vi "Create Listbox IP Text - Multi FPGA.vi"(8 "error in (no error)":errorcluster, 10 "rios and analog replays":T1(array[cluster]), 11 "Section Ref in":T2 format="%.0x") -> (0 "error out":errorcluster, 2 "listbox text":string[][](array[string]), 3 "Section Ref out":T2 format="%.0x", 5 "not present item indexes":i32[](array[numeric]))   [LabVIEW 2015, in "Engine Simulation Toolkit System Explorer.lvlib"]
uses:
  Engine Simulation Toolkit System Explorer.lvlib
  <vilib>/NI Veristand/Custom Device API/Custom Device Item Ref.ctl
  Shared/Properties.vi
  Shared/Constants and GUIDs.vi
  <vilib>/NI Veristand/Custom Device API/Get Item Property (String).vi
  <vilib>/NI Veristand/Custom Device API/Custom Device API.lvlib
  Shared/Engine Simulation Toolkit Shared.lvlib
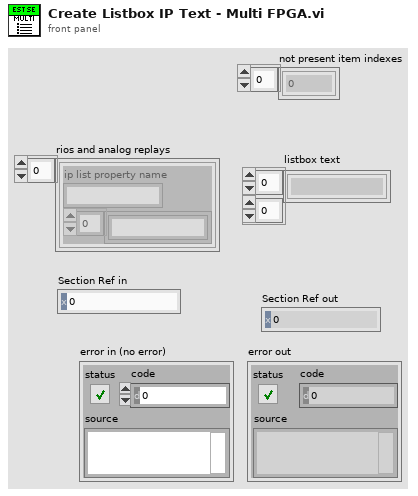
[diagram p1: front panel]
types:
  T1 = cluster{"ip list property name":string, string[]}[]
  T2 = typedef "Custom Device API.lvlib/Custom Device Item Ref.ctl" = u64
  T3 = typedef "Custom Device API.lvlib/Custom Device Item Info.ctl" = cluster{"Name":string, "Is Channel":bool, "GUID":string, "Is Waveform":bool}
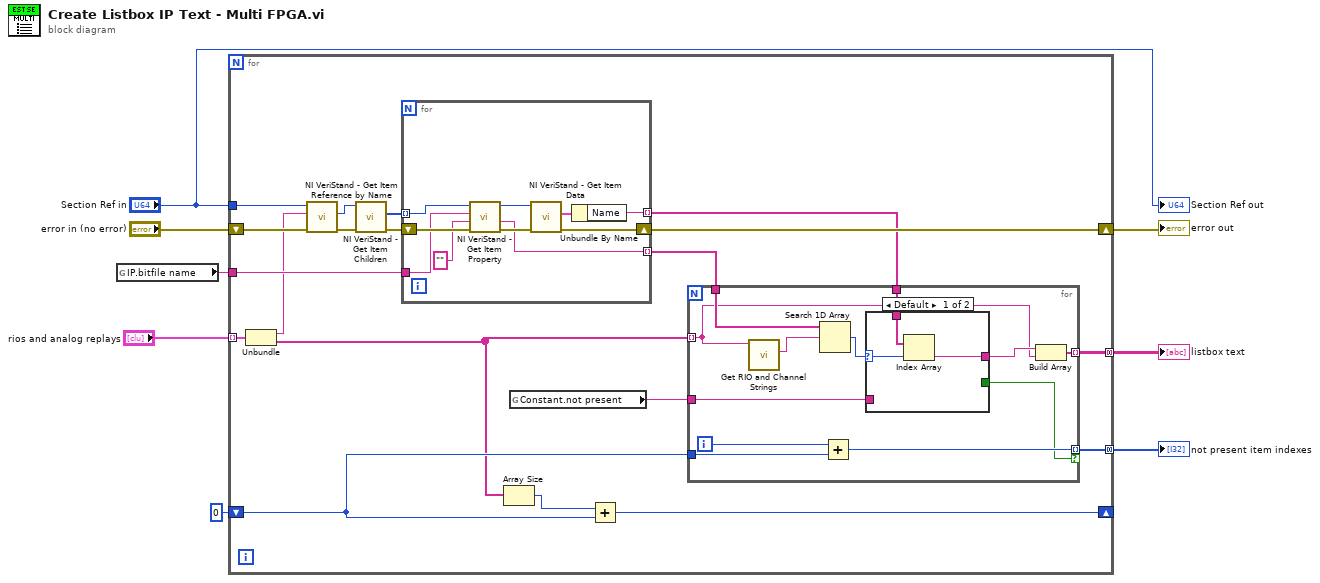
[diagram p0: block diagram]
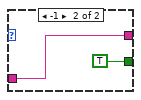
[diagram p2: hidden frame]
diagram:
  n1 = global read "Properties.vi" "IP.bitfile name"() -> (w8:string)
  n2 = for {
    tunnel: w8 -> [w27]
    tunnel: "rios and analog replays" -> [w18] mode=indexing
    tunnel: [w21] -> w7 mode=concatenating
    tunnel: [w24] -> w6 mode=concatenating
    shift-right: [w26] -> w1
    shift-left: "error in (no error)" -> [w16]
    shift-right: [w20] -> _
    shift-left: 0 -> [w19]
    tunnel: "Section Ref in" -> [w15]
    n3 = Unbundle(w18) -> ("ip list property name"=w14:string, w9:string[])
    n4 = call <vilib>:"NI VeriStand - Get Item Reference by Name.vi"("error in (no error)"=w16, "Item Name"=w14, "Parent Ref in"=w15) -> ("error out"=w17:errorcluster, "Item Ref"=w11:T2)  [unwired: 5 in, 2 out]
    n5 = call <vilib>:"NI VeriStand - Get Item Children.vi"("error in (no error)"=w17, "Item Ref in"=w11) -> ("error out"=w22:errorcluster, "Child Refs"=w23:T2[])  [unwired: 6 in, 2 out]
    n6 = for {
      shift-right: [w49] -> w26
      shift-left: w22 -> [w54]
      tunnel: w23 -> [w52] mode=indexing
      tunnel: w27 -> [w51]
      tunnel: [w46] -> w13 mode=indexing
      tunnel: [w45] -> w12 mode=indexing
      n7 = call-poly <vilib>:"NI VeriStand - Get Item Property.vi"("error in (no error)"=w54, "Default Value"="", "Property Name"=w51, "Item Ref in"=w52) -> ("error out"=w53:errorcluster, "Value"=w46:string, "Item Ref out"=w48:T2)  [unwired: 4 in, 1 out]
      n8 = call <vilib>:"NI VeriStand - Get Item Data.vi"("error in (no error)"=w53, "Item Ref in"=w48) -> ("error out"=w49:errorcluster, "Item Info"=w47:T3)  [unwired: 6 in, 2 out]
      n9 = Unbundle By Name(w47) -> ("Name"=w45:string)
    }
    n10 = Array Size(array=w9) -> (size(s)=w10:i32)
    n11 = global read "Constants and GUIDs.vi" "Constant.not present"() -> (w25:string)
    n12 = Add(x=w10, y=w19) -> (x+y=w20:i32)
    n13 = for {
      tunnel: w9 -> [w29] mode=indexing
      tunnel: w13 -> [w39]
      tunnel: w12 -> [w37]
      tunnel: [w35] -> w21 mode=indexing
      tunnel: w25 -> [w34]
      tunnel: [w31] -> w24 mode=indexing if=w30
      tunnel: w19 -> [w32]
      i -> [w33]
      n14 = call "Get RIO and Channel Strings.vi"("rio/channel"=w29) -> ("channel"=w28:string)  [unwired: 9 in, 1 out]
      n15 = Search 1D Array(1D array=w39, element=w28) -> (index of element=w38:i32)  [unwired: 1 in]
      n16 = Add(x=w33, y=w32) -> (x+y=w31:i32)
      n17 = case shown="Default" w38 {
        selector: w38 -> [w41 _]
        tunnel: [w40 w44] -> w36
        tunnel: w37 -> [w42 _]
        tunnel: w34 -> [_ w44]
        tunnel: [_ TRUE] -> w30
        frame Default {
          n18 = Index Array(array=w42, index=w41) -> (element=w40:string)
        }
        frame -1 {
        }
      }
      n19 = Build Array(w36, w29) -> (w35:string[])
    }
  }
  "error out" <- w1
  "listbox text" <- w7
  "not present item indexes" <- w6
  "Section Ref out" <- "Section Ref in"
